vi "false if multiple false.vi"(8 "Max elements":i64=100, 11 "Fail":bool) -> (3 "Multiple fail":bool)   [LabVIEW 2015]
panel:
  out "Array":bool[](array[boolean])
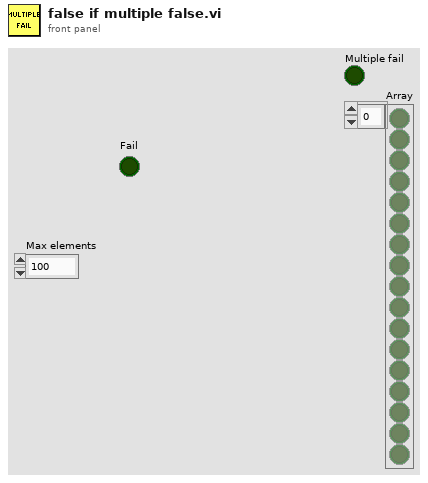
[diagram p1: front panel]
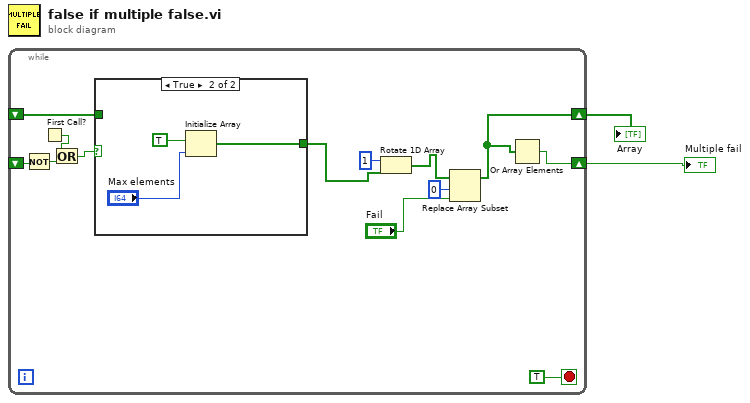
[diagram p0: block diagram]
diagram:
  n1 = while {
    shift-right: [w8] -> w2
    shift-left: _ -> [w14]
    shift-right: [w7] -> w1
    shift-left: _ -> [w6]
    stop <- TRUE stop-if-true
    n2 = Not(x=w6) -> (.not. x?=w5:bool)
    n3 = First Call?() -> (First Call?: T/F=w4:bool)
    n4 = Or(x=w4, y=w5) -> (x .or. y?=w3:bool)
    n5 = case shown="True" w3 {
      tunnel: [w16 w17] -> w13
      tunnel: w14 -> [w16 _]
      frame False {
      }
      frame True {
        n6 = Initialize Array(TRUE ("Fail"), "Max elements") -> (w17:bool[])
      }
    }
    n7 = Rotate 1D Array(1:w13, 2:1 ("n")) -> (0:w11:bool[])
    n8 = Replace Array Subset(array=w11, new element="Fail", index=0) -> (w8:bool[])
    n9 = Or Array Elements(Boolean array=w8) -> (logical OR=w7:bool)
  }
  "Multiple fail" <- w1
  "Array" <- w2
